vi "DigitalInput Event Example.vi"() -> ()   [LabVIEW 2012, in "Phidget Digital Input.lvlib"]
uses:
  <instrlib>/Phidgets/Phidget Digital Input/Phidget Digital Input.lvlib
  <instrlib>/Phidgets/Phidget Digital Input/Public/DigitalInputStart.vi
  <instrlib>/Phidgets/Phidget Digital Input/Public/DigitalInputClose.vi
  <instrlib>/Phidgets/Phidget Common/Phidget Common.lvlib
panel:
  in  "Is Hub Port?":bool
  out "State":bool
  in  "stop":bool
  out "Serial Number Return":i32
  in  "Device Info":T1={"Serial Number"=-1, "Channel"=0, "Port"=0}
  out "error out":errorcluster
  # "Be sure to use this stop button to stop the program.\nIf you use the \"Abort Execution\" button, you will\nneed to use PhidgetResetLibrary.vi or restart Labview \nin order for any Phidgets to work."
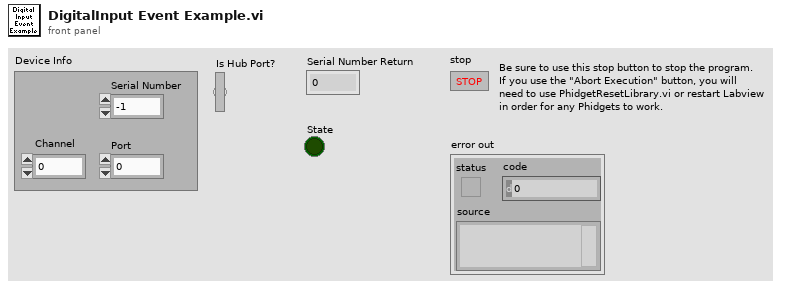
[diagram p1: front panel]
types:
  T1 = cluster{"Serial Number":i32, "Channel":i32, "Port":i32}
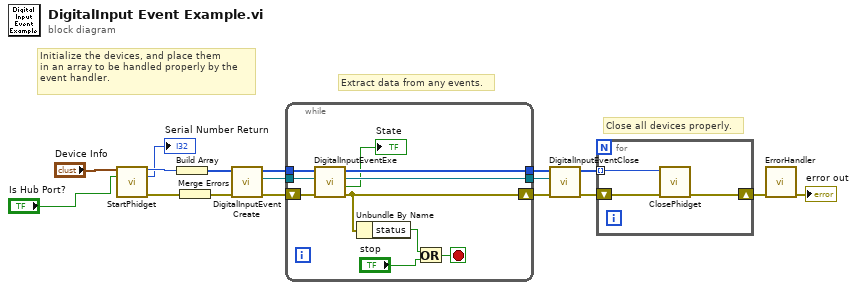
[diagram p0: block diagram]
diagram:
  # "Close all devices properly."
  # "Extract data from any events."
  # "Initialize the devices, and place them\nin an array to be handled properly by the\nevent handler."
  n1 = call-poly <instrlib>:"StartPhidget.vi"("Device Info"="Device Info", "IsHubPort"="Is Hub Port?") -> ("Phidget ID"=w6:u64, "Serial Number Return"=→"Serial Number Return":i32, "error out"=w1:errorcluster)  [unwired: 10 in, 1 out]
  n2 = Build Array(w6) -> (w17:u64[])
  n3 = Merge Errors(w1) -> (w8:errorcluster)
  n4 = call <instrlib>:"DigitalInputEventCreate.vi"("error in (no error)"=w8, "Devices In"=w17) -> ("error out"=w10:errorcluster, "Event Registration Refnum"=w15:refnum<event-registration>, "Devices Out"=w16:u64[])  [unwired: 7 in]
  n5 = while {
    tunnel: w16 -> [w27]
    tunnel: w15 -> [w23]
    tunnel: [w26] -> w12
    shift-right: [w22] -> w11
    shift-left: w10 -> [w25]
    tunnel: [w24] -> w4
    stop <- w21 stop-if-true
    n6 = call <instrlib>:"DigitalInputEventExe.vi"("error in (no error)"=w25, "Event Registration Refnum In"=w23, "Devices In"=w27) -> ("error out"=w22:errorcluster, "State"=→"State":bool, "Event Registration Refnum Out"=w26:refnum<event-registration>, "Devices Out"=w24:u64[])  [unwired: 1 in, 4 out]
    n7 = Unbundle By Name(w22) -> ("status"=w19:bool)
    n8 = Or(x=w19, y="stop") -> (x .or. y?=w21:bool)
  }
  n9 = call <instrlib>:"DigitalInputEventClose.vi"("error in (no error)"=w11, "Event Registration Refnum In"=w12, "Devices In"=w4) -> ("error out"=w7:errorcluster, "Devices Out"=w5:u64[])  [unwired: 7 in]
  n10 = for {
    tunnel: w5 -> [w28] mode=indexing
    shift-right: [w30] -> w14
    shift-left: w7 -> [w29]
    n11 = call-poly <instrlib>:"ClosePhidget.vi"("error in"=w29, "Device In"=w28) -> ("error out"=w30:errorcluster)  [unwired: 9 in]
  }
  n12 = call <instrlib>:"ErrorHandler.vi"("error in"=w14) -> ("error out"=→"error out":errorcluster)  [unwired: 9 in, 1 out]
